vi "TranslateRequestTopic.vi"(2 "String w/o Tag":string, 3 "Registered":T2[](array[typedef])) -> (0 "XML":string, 1 "New Sub":T1)   [LabVIEW 2016]
doc: "Returns the port or if the port already exists, make up a new one and then add that to the publisher queue"
uses:
  _ROSControl.ctl
  _ROSDirection.ctl
panel:
  out "topic port":u16
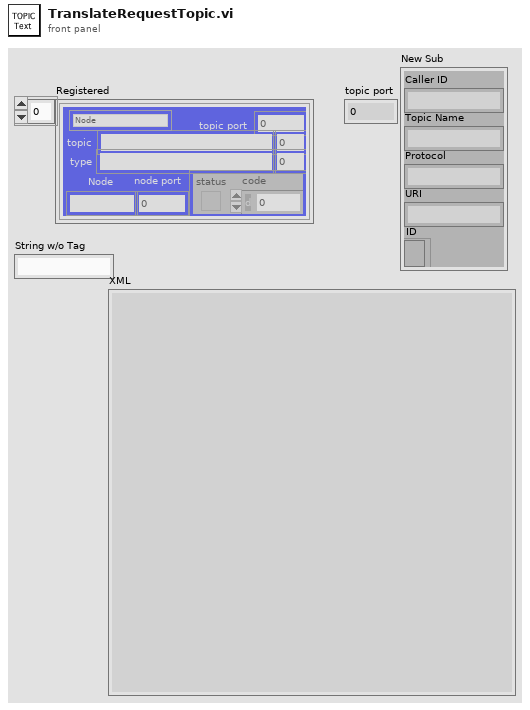
[diagram p1: front panel]
types:
  T1 = cluster{"Caller ID":string, "Topic Name":string, "Protocol":string, "URI":string, "ID":refnum<k5>}
  T2 = typedef "_ROSControl.ctl" = cluster{"topic port":u16, "Node":string, "topic":string, "type":string, "node port":u16, "error ":errorcluster, "Direction":T3, "Update (ms)":u16, "FIFO size":u16}
  T3 = typedef "_ROSDirection.ctl" = enum16{"Node", "Publisher", "Subscriber", "ServiceClient", "ServiceProvider"}
  T4 = enum16{"rosrpc://IP:port", "http://IP:port", "http://IP", "IP:port", "IP only"}
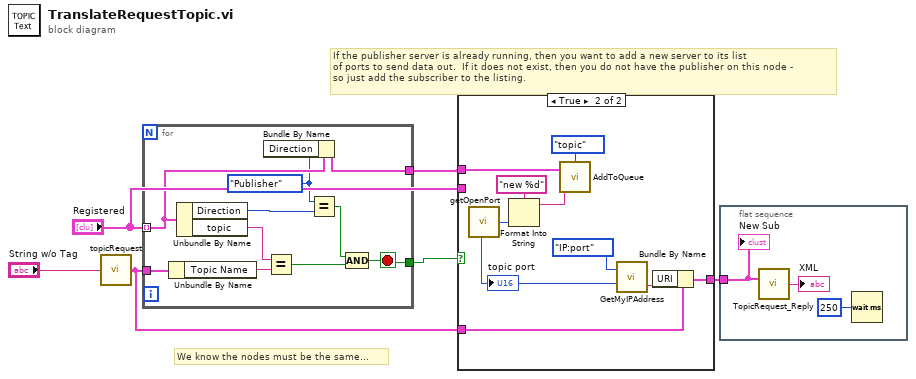
[diagram p0: block diagram]
diagram:
  # "If the publisher server is already running, then you want to add a new server to its list\nof ports to send data out.  If it does not exist, then you do not have the publisher on this node - \nso just add the subscriber to the listing."
  # "We know the nodes must be the same..."
  n1 = call "topicRequest.vi"("XML"="String w/o Tag") -> ("Subscriber"=w5:T1)
  n2 = for {
    tunnel: "Registered" -> [w9] mode=indexing
    tunnel: w5 -> [w16]
    tunnel: [w10] -> w3
    tunnel: [w7] -> w1
    stop <- w10 stop-if-true
    w8 = _ROSDirection."Publisher" ("x")
    n3 = Unbundle By Name(w16) -> ("Topic Name"=w15:string)
    n4 = Unbundle By Name(w9) -> ("Direction"=w13:T3, "topic"=w14:string)
    n5 = Bundle By Name(cluster=w9, "Direction"=w8) -> (w7:T2)
    n6 = Equal?(x=w14, y=w15) -> (x = y?=w11:bool)
    n7 = Equal?(x=w8, y=w13) -> (x = y?=w12:bool)
    n8 = Compound Arithmetic op=AND(w12, w11) -> (w10:bool)
  }
  n9 = case shown="True" w3 {
    tunnel: w5 -> [w17 w21]
    tunnel: [w17 w20] -> w4
    tunnel: "Registered" -> [_ _]
    tunnel: w1 -> [_ w23]
    frame False {
    }
    frame True {
      n10 = call "getOpenPort.vi"() -> ("port"=w24:u16)
      "topic port" <- w24
      n11 = Format Into String(format string="new %d", w24) -> (resulting string=w22:string)  [unwired: 2 in, 1 out]
      n12 = call "AddToQueue.vi"("Cmd"=w22, "ROS"=w23, "Type"=enum16{"topic", "node", "ToFIFO", "ToWrite"}."topic") -> ()  [unwired: 2 in, 1 out]
      n13 = call "GetMyIPAddress.vi"("Port"=w24, "Format"=T4."IP:port") -> ("URI"=w26:string)  [unwired: 1 out]
      n14 = Bundle By Name(cluster=w21, "URI"=w26) -> (w20:T1)
    }
  }
  n15 = flat-sequence {
    tunnel: w4 -> [w29]
    frame #0 {
      n16 = call "TopicRequest_Reply.vi"("Subscriber"=w29) -> ("XML"=→"XML":string)  [unwired: 1 in]
      n17 = Wait (ms)(milliseconds to wait=u32 250) -> ()  [unwired: 1 out]
      "New Sub" <- w29
    }
  }
